vi "WT-Voltage-Controller-Current.vi"() -> ()   [LabVIEW 2017]
uses:
  <vilib>/Platform/TimedLoop/XDataNode/timing_clust.ctl
  <vilib>/Platform/TimedLoop/XDataNode/nitl_modes.ctl
  <vilib>/Platform/TimedLoop/XDataNode/wakeup.ctl
  <vilib>/DAQmx/read.llb/DAQmx Read (Analog 1D DBL NChan 1Samp).vi
  <vilib>/Analysis/baseanly.llb/Mean (DBL).vi
  <vilib>/DAQmx/miscellaneous.llb/DAQmx Fill In Error Info.vi
  <vilib>/express/express shared/transition.llb/Dynamic To Waveform Array.vi
  <vilib>/express/express signal manip/GetorSetDDTAttributes/Set DDT Attributes/SetT0.vi
  <vilib>/express/express shared/transition.llb/Waveform Array To Dynamic.vi
  <vilib>/platform/TimedLoop/XDataNode/XDataNode.xnode
  <vilib>/express/express signal manip/GetorSetDDTAttributes/Set DDT Attributes/Set DDT Properties.xnode
  <vilib>/Platform/TimedLoop/XDataNode/XDNodeRunTimeDep.lvlib
  <vilib>/Analysis/NI_AALBase.lvlib
panel:
  out "Fan 2 (A)":dbl format="%0.2f"
  out "Fan 1 (A)":dbl format="%0.2f"
  out "Boolean":bool
  in  "POWER":bool
  in  "Sync":bool
  out "error out":errorcluster
  in  "Fan 2 Voltage":dbl(knob) scale=0.0..10.0
  in  "Fan 1 Voltage":dbl(knob) scale=0.0..10.0
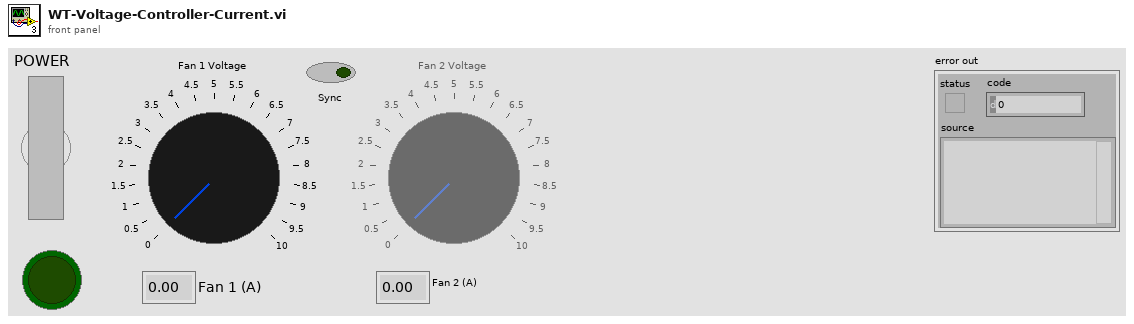
[diagram p1: front panel]
types:
  T1 = typedef "XDNodeRunTimeDep.lvlib/timing_clust.ctl" = cluster{"Expected End [f-1]":u64, "Actual End [f-1]":u64, "Finished Late? [f-1]":bool, "Expected End [i-1]":u64, "Actual End [i-1]":u64, "Finished Late? [i-1]":bool, "Expected Start [i]":u64, "Actual Start [i]":u64, "Expected Start [f]":u64, "Actual Start [f]":u64, "Source Name":string, "Structure Name":string, "Period":i64, "Deadline":i64, "Offset":i64, "Start":i64, "Priority":i32, "Timeout":i32, "Mode":T2, "Wakeup Reason":T3, "Error":errorcluster, "Source Type":string, "Secondary Source Type":string, "Global End Time":u64, "Global Start Time":u64, "Frame Duration":u64, "Iteration Duration":u64, "Assigned CPU":i32, "I/O Scan Engine Mode":u32}
  T2 = typedef "XDNodeRunTimeDep.lvlib/nitl_modes.ctl" = enum32{"No Change", "Process missed periods, maintain original phase", "Discard missed periods, maintain original phase", "Process missed periods, ignore original phase", "Discard missed periods, ignore original phase"}
  T3 = typedef "XDNodeRunTimeDep.lvlib/wakeup.ctl" = enum32{"Normal", "Aborted", "Asynchronous wakeup", "Timing source error", "Timed loop error", "Timeout"}
  T4 = enum8{"Enabled", "Disabled", "Disabled and Grayed Out"}
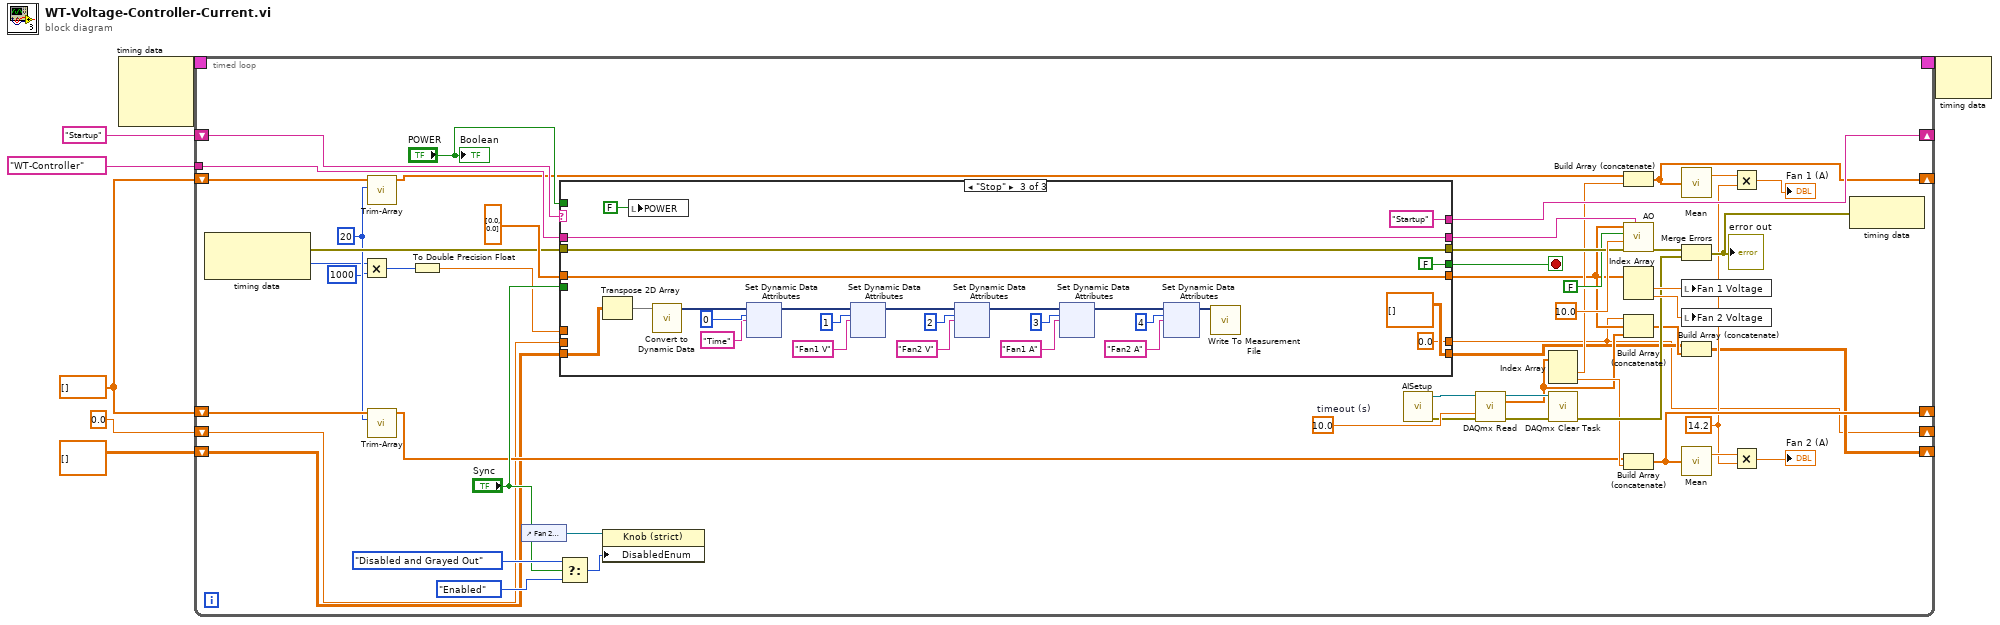
[diagram p0: block diagram]
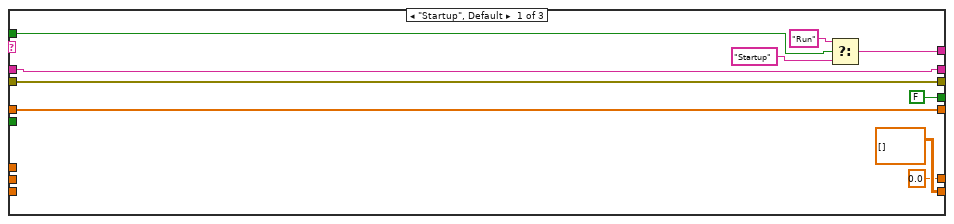
[diagram p2: hidden frame]
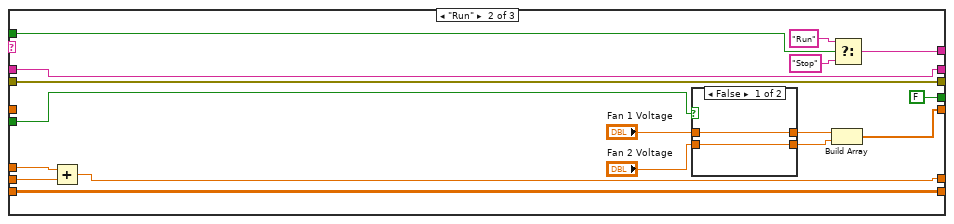
[diagram p3: hidden frame]
diagram:
  w3 = dbl[] []
  n1 = node-c288() -> (w5:T1)  [unwired: 3 in]
  n2 = timed-loop {
    shift-right: [w58] -> _
    shift-left: "Startup" -> [w59]
    tunnel: tag "WT-Controller" ("device name") -> [w56]
    timing: w5 -> [_]
    timing-out: [_] -> w4
    shift-right: [w30] -> _
    shift-left: w3 -> [w28]
    shift-right: [w29] -> _
    shift-left: w3 -> [w27]
    shift-right: [w16] -> _
    shift-left: dbl[][] [] -> [w14]
    shift-right: [w8] -> _
    shift-left: 0.0 -> [w10]
    stop <- w57 stop-if-true
    w21 = 14.2 ("y")
    w25 = 20 ("length")
    w41 = 10.0  # timeout (s)
    n3 = node-c288() -> (w46:errorcluster, w13:i64)  [unwired: 1 in]
    n4 = Multiply(x=w13, y=i64 1000) -> (x*y=w11:i64)
    n5 = call "Trim-Array.vi"("length"=w25, "Array in"=w28) -> ("Array out"=w32:dbl[])  [unwired: 9 in]
    n6 = call "Trim-Array.vi"("length"=w25, "Array in"=w27) -> ("Array out"=w26:dbl[])  [unwired: 9 in]
    n7 = To Double Precision Float(number=w11) -> (double precision float=w9:dbl)
    n8 = control-ref of="Fan 2 Voltage"() -> (w52:refnum<vi>)
    n9 = case shown="\"Stop\"" w59 {
      tunnel: [w69 w92 "Startup" ("f")] -> w58
      tunnel: [w74 w85 w119] -> w19
      tunnel: [FALSE ("Stop") FALSE ("Stop") FALSE ("Stop")] -> w57
      tunnel: w56 -> [w73 w84 w120]
      tunnel: [w75 w83 w118] -> w48
      tunnel: w46 -> [w75 w83 w118]
      tunnel: "Sync" -> [_ w87 _]
      tunnel: dbl[] [0.0, 0.0] ("appended array") -> [w74 _ w119]
      tunnel: [w73 w84 w120] -> w47
      tunnel: "POWER" -> [w71 w82 _]
      tunnel: [dbl[][] [] w79 dbl[][] []] -> w15
      tunnel: w14 -> [_ w79 w114]
      tunnel: w10 -> [_ w78 _]
      tunnel: [0.0 w76 0.0] -> w8
      tunnel: w9 -> [_ w77 _]
      frame "Startup", Default {
        n10 = Select(t="Run" ("f"), s=w71, f="Startup") -> (s? t:f=w69:string)
      }
      frame "Run" {
        n11 = Add(x=w77, y=w78) -> (x+y=w76:dbl)
        n12 = case shown="False" w87 {
          tunnel: [w93 w95] -> w90
          tunnel: [w94 w95] -> w89
          tunnel: "Fan 1 Voltage" -> [w94 w95]
          tunnel: "Fan 2 Voltage" -> [w93 _]
          frame False {
          }
          frame True {
          }
        }
        n13 = Build Array(w89, w90) -> (w85:dbl[])
        n14 = Select(t="Run" ("f"), s=w82, f="Stop") -> (s? t:f=w92:string)
      }
      frame "Stop" {
        n15 = Transpose 2D Array(2D array=w114) -> (transposed array=w112:dbl[][])
        n16 = local write "POWER"(FALSE ("POWER")) -> ()
        n17 = call "Convert to Dynamic Data"("2D Array"=w112) -> ("Dynamic Data Type"=w113:dynamicdata)  [unwired: 3 in]
        n18 = xnode ("Set Dynamic Data Attributes")("Signals In"=w113, "Signal Index"=0, "Signal Name"="Time") -> ("Signals Out"=w108:dynamicdata)  [unwired: 1 in, 1 out]
        n19 = xnode ("Set Dynamic Data Attributes")("Signals In"=w108, "Signal Index"=1, "Signal Name"="Fan1 V") -> ("Signals Out"=w105:dynamicdata)  [unwired: 1 in, 1 out]
        n20 = xnode ("Set Dynamic Data Attributes")("Signals In"=w105, "Signal Index"=2, "Signal Name"="Fan2 V") -> ("Signals Out"=w104:dynamicdata)  [unwired: 1 in, 1 out]
        n21 = xnode ("Set Dynamic Data Attributes")("Signals In"=w104, "Signal Index"=3, "Signal Name"="Fan1 A") -> ("Signals Out"=w101:dynamicdata)  [unwired: 1 in, 1 out]
        n22 = xnode ("Set Dynamic Data Attributes")("Signals In"=w101, "Signal Index"=4, "Signal Name"="Fan2 A") -> ("Signals Out"=w100:dynamicdata)  [unwired: 1 in, 1 out]
        n23 = call "Write To Measurement File"("Signals"=w100) -> ()  [unwired: 16 in, 3 out]
      }
    }
    n24 = Select(t=T4."Disabled and Grayed Out" ("Disabled"), s="Sync", f=T4."Enabled") -> (s? t:f=w54:T4)
    n25 = property class="Knob (strict)"(reference=w52, "DisabledEnum"=w54) -> ()  [unwired: 1 in, 2 out]
    n26 = call "AISetup.vi"() -> ("error out"=w37:errorcluster, "task out"=w38:refnum<k21>)  [unwired: 10 in]
    n27 = call-poly <vilib>:"DAQmx Read.vi"("task/channels in"=w38, "timeout"=w41, "error in"=w37) -> ("task out"=w39:refnum<k21>, "data"=w18:dbl[], "error out"=w40:errorcluster)  [unwired: 10 in]
    n28 = Index Array(array=w18) -> (element #1=w33:dbl, element #2=w31:dbl)  [unwired: 2 in]
    n29 = call <vilib>:"DAQmx Clear Task.vi"("task in"=w39, "error in"=w40) -> ("error out"=w36:errorcluster)  [unwired: 13 in]
    n30 = Build Array (concatenate)(w32, w33) -> (w30:dbl[])
    n31 = call "AO.vi"("device name"=w47, "error in"=w48, "timeout (s)"=10.0, "stop (T)"=FALSE, "data"=w19) -> ("error out"=w35:errorcluster)  [unwired: 2 in, 1 out]
    n32 = Index Array(array=w19) -> (element #1=w45:dbl, element #2=w44:dbl)  [unwired: 2 in]
    n33 = Build Array (concatenate)(w8, w19, w18) -> (w17:dbl[])
    n34 = Build Array (concatenate)(w26, w31) -> (w29:dbl[])
    n35 = call-poly <vilib>:"Mean.vi"("X"=w30) -> ("mean"=w24:dbl)  [unwired: 1 out]
    n36 = Merge Errors(w35, w36) -> (w34:errorcluster)
    "error out" <- w34
    n37 = local write "Fan 1 Voltage"(w45) -> ()
    n38 = local write "Fan 2 Voltage"(w44) -> ()
    n39 = Build Array (concatenate)(w15, w17) -> (w16:dbl[][])
    n40 = call-poly <vilib>:"Mean.vi"("X"=w29) -> ("mean"=w22:dbl)  [unwired: 1 out]
    n41 = Multiply(x=w24, y=w21) -> (x*y=→"Fan 1 (A)":dbl)
    n42 = Multiply(x=w22, y=w21) -> (x*y=→"Fan 2 (A)":dbl)
    n43 = node-c288(w34) -> ()  [unwired: 1 out]
    "Boolean" <- "POWER"
  }
  n44 = node-c288(w4) -> ()  [unwired: 1 out]
